vi "Configure Output Range.vi"(8 "error in (no error)":errorcluster, 10 "Voltage Range (0: Low)":u16(ring) items=["Low", "High"], 11 "VISA resource name":refnum<visa-resource-name>) -> (0 "error out":errorcluster, 3 "VISA resource name out":refnum<visa-resource-name>)   [LabVIEW 2009, in "Agilent E363X Series.lvlib"]
doc: "Configures the voltage range. \n\n<B>Note:</B> Not supported on E3631"
uses:
  <instrlib>/Agilent E363X Series/Agilent E363X Series.lvlib
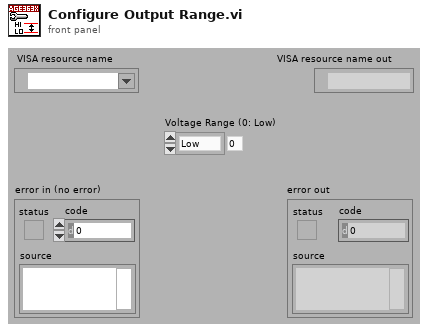
[diagram p1: front panel]
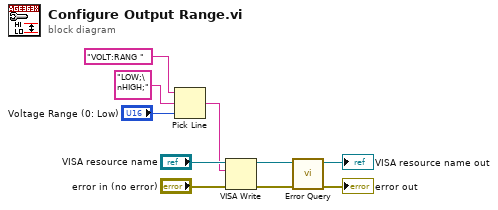
[diagram p0: block diagram]
diagram:
  n1 = Pick Line(string ("")="VOLT:RANG " ("initial string"), multi-line string="LOW;\nHIGH;" ("true string"), line index="Voltage Range (0: Low)") -> (output string=w7:string)
  n2 = VISA Write(VISA resource name="VISA resource name", write buffer=w7, error in (no error)="error in (no error)") -> (VISA resource name out=w5:refnum<visa-resource-name>, error out=w6:errorcluster)  [unwired: 1 out]
  n3 = call <instrlib>:"Error Query.vi"("error in (no error)"=w6, "VISA resource name"=w5) -> ("error out"=→"error out":errorcluster, "VISA resource name out"=→"VISA resource name out":refnum<visa-resource-name>)  [unwired: 6 in, 2 out]
